vi "Get Audit Trail Data.vi"(8 "error in (no error)":errorcluster, 11 "file path (dialog if empty)":path) -> (0 "error out":errorcluster, 3 "all rows":string[][](array[string]))   [LabVIEW 2025]
uses:
  <vilib>/Utility/file.llb/Read Delimited Spreadsheet (string).vi
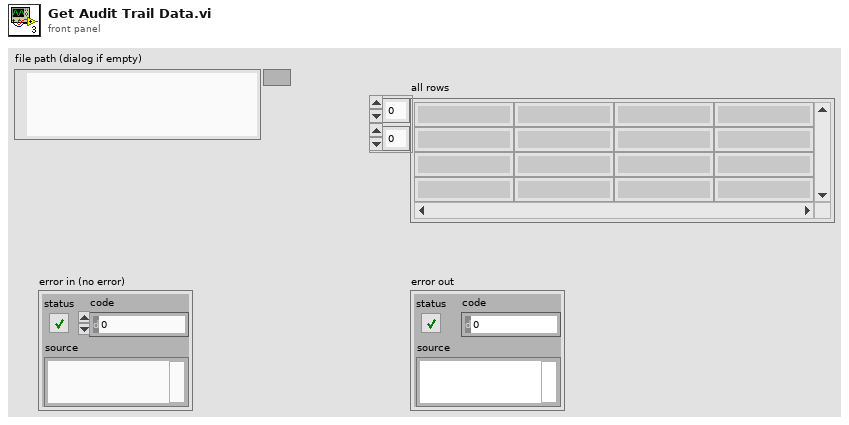
[diagram p1: front panel]
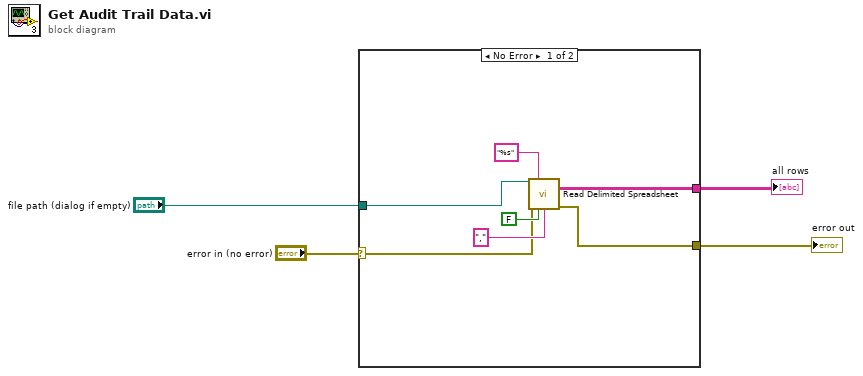
[diagram p0: block diagram]
diagram:
  n1 = case shown="No Error" "error in (no error)" {
    selector: "error in (no error)" -> [w6 w12]
    tunnel: [w11 w12] -> w4
    tunnel: [w9 _] -> w3
    tunnel: "file path (dialog if empty)" -> [w5 _]
    frame No Error {
      n2 = call-poly <vilib>:"Read Delimited Spreadsheet.vi"("file path (dialog if empty)"=w5, "format (%s)"="%s", "error in (no error)"=w6, "transpose? (F)"=FALSE, "delimiter (\\t)"="," ("delimiter (\\t)")) -> ("all rows"=w9:string[][], "error out"=w11:errorcluster)  [unwired: 5 in, 4 out]
    }
    frame Error {
    }
  }
  "error out" <- w4
  "all rows" <- w3
